vi "AlliGator Update Background Subtraction Indicators.vi"(8 "Error In":errorcluster, 10 "Decay Metadata":T1={"ROI Descriptor"={"Global Rectangle"=[], "Contours"=[]}, "ROI Center"={"X"=0, "Y"=0}, "Decay Background Subtraction Info"={"Laser Period"=0.0, "Gate Duration"=0.0, "Baseline Subtraction Method"=enum."Mean", "Background Definition Range"={"Min Gate"=0.0, "Max Gate"=0.0}, "Total Intensity w/o Bkgd Subtraction"=0.0, "Bkgd-subtracted Intensity (exp)"=0.0, "# Data Points"=0, "Background/Gate"=0.0, "Fitted Lifetime"=0.0, "Bkgd-subtracted Intensity (theo)"=0.0}, "Decay Reverted"=FALSE, "Decay Smoothened"=FALSE, "Decay Straightened"=FALSE, "Fitted Tau (Decay Straightening)"=0.0, "Decay Shift Parameters"={"Type"=enum."Default", "Shift"=0.0, "Threshold"=0.0, "Rotate"=FALSE}, "Decay Shifted"=FALSE, "Decay Extrapolated"=FALSE, "Decay Extrapolation Parameters"={"Additional Points"=0, "Head Fraction"=0.0, "Fitted Tau"=0.0, "Use Periodicity"=FALSE, "Use Cursors"=FALSE, "Tail Fraction"=0.0}, "Decay Normalized"=FALSE, "Fold Decay"=FALSE, "# Folds"=1} {"# Folds" min=1; "ROI Descriptor"."Contours"."Type" items=["No Selection", "Point", "Line", "Rectangle", "Oval", "Polygon", "Freehand Region", "Annulus", "Unused2", "Unused3", "Broken Line", "Freehand Line", "Rotated Rectangle"]}, 11 "AlliGator Ref":refnum<vi>) -> (0 "Error Out":errorcluster)   [LabVIEW 2021, in "AlliGator Decay Analysis.lvlib" / "AlliGator Decay Preprocessing.lvlib"]
doc: "Updates background subtraction indicators in the <B>Decay Graph</B> panel."
uses:
  AlliGator Decay Preprocessing.lvlib
  AlliGator Decay Metadata v3.ctl
  AlliGator Decay Background Subtraction Info.ctl
  AlliGator Baseline Subtraction Method.ctl
  Graphs/XY Graph/XY Graph Plot Shift Parameters.ctl
  Graphs/XY Graph/XY Graph Plot Shift Method.ctl
  AlliGator Decay Extrapolation Parameters.ctl
  AlliGator Settings List.ctl
  Variant/Variant to Data/Variant to Boolean.vi
  AlliGator Settings.lvlib
  Variant/Variant to Data/Variant to Data.lvlib
  Utilities/Utilities.lvlib
  AlliGator Phasor Graph.lvlib
  Graphs/XY Graph/XY Graph Add-Ons.lvlib
panel:
  out "Integrated Intensity":dbl
  out "Lifetime":dbl[unit]=nan
  out "Background/Gate":dbl
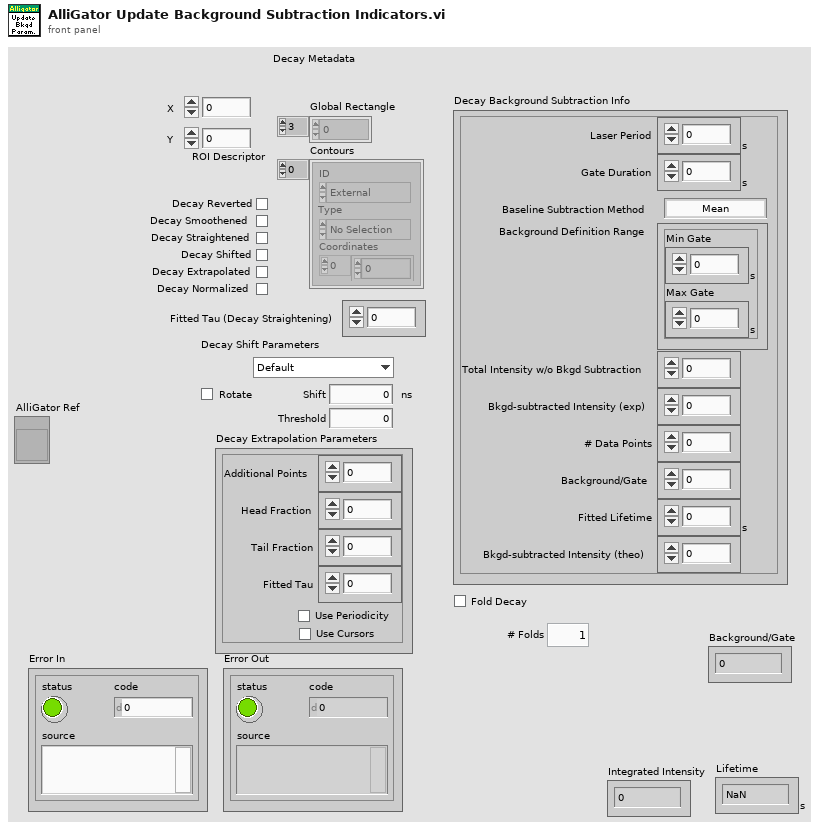
[diagram p1: front panel]
types:
  T1 = typedef "AlliGator Phasor Graph.lvlib/AlliGator Decay Metadata v3.ctl" = cluster{"ROI Descriptor":T2, "ROI Center":cluster{"X":i32, "Y":i32}, "Decay Background Subtraction Info":T3, "Decay Reverted":bool, "Decay Smoothened":bool, "Decay Straightened":bool, "Fitted Tau (Decay Straightening)":dbl, "Decay Shift Parameters":T5, "Decay Shifted":bool, "Decay Extrapolated":bool, "Decay Extrapolation Parameters":T7, "Decay Normalized":bool, "Fold Decay":bool, "# Folds":u32}
  T2 = typedef "ROI Descriptor" = cluster{"Global Rectangle":i32[], "Contours":cluster{"ID":enum32{"External", "Internal"}, "Type":u32, "Coordinates":i32[]}[]}
  T3 = typedef "AlliGator Decay Analysis.lvlib/AlliGator Decay Preprocessing.lvlib/AlliGator Decay Background Subtraction Info.ctl" = cluster{"Laser Period":dbl[unit], "Gate Duration":dbl[unit], "Baseline Subtraction Method":T4, "Background Definition Range":cluster{"Min Gate":dbl[unit], "Max Gate":dbl[unit]}, "Total Intensity w/o Bkgd Subtraction":dbl, "Bkgd-subtracted Intensity (exp)":dbl, "# Data Points":i32, "Background/Gate":dbl, "Fitted Lifetime":dbl[unit], "Bkgd-subtracted Intensity (theo)":dbl}
  T4 = typedef "AlliGator Decay Analysis.lvlib/AlliGator Decay Preprocessing.lvlib/AlliGator Baseline Subtraction Method.ctl" = enum16{"Mean", "Min", "Square Gated Single-Exponential", "File", "Constant"}
  T5 = typedef "XY Graph Add-Ons.lvlib/XY Graph Plot Shift Parameters.ctl" = cluster{"Type":T6, "Shift":dbl[unit], "Threshold":dbl, "Rotate":bool}
  T6 = typedef "XY Graph Add-Ons.lvlib/XY Graph Plot Shift Method.ctl" = enum16{"Default", "CFD", "Threshold", "Cross-Correlation"}
  T7 = typedef "AlliGator Decay Analysis.lvlib/AlliGator Decay Preprocessing.lvlib/AlliGator Decay Extrapolation Parameters.ctl" = cluster{"Additional Points":u32, "Head Fraction":dbl, "Fitted Tau":dbl, "Use Periodicity":bool, "Use Cursors":bool, "Tail Fraction":dbl}
  T8 = typedef "AlliGator Settings.lvlib/AlliGator Settings List.ctl" = enum16{"GUI:Visible Settings Tab", "GUI:Last Run Version", "Source Image:Use Image Histogram for Contrast", "Source Image:Low Count Pixels Rejection Options", "Source Image:High Count Pixels Rejection Options", "Source Image:Use Image Brightness", "Source Image:Blend Overlay with Image Background", "Source Image:Use Fixed ROI Diameter", "Source Image:ROI Diameter", "Source Image:ROI Center Color", "Source Image:Peak Threshold", "Source Image:Intensity Threshold", "Source Image:Image Binning Options", "Source Image:Image Smoothing Options", "Source Image:Image Histogram Active", "Source Image:Invert Binary Mask", "Source Image:Hot Pixel Removal", "Source Image:Overlay Analyzed ROI Center", "Source Image:Auto-Adjust Contrast", "Source Image:Histogram Lower Percentile", "Source Image:Histogram Upper Percentile", "Source Image:Save Source Image", "Source Image:Scale Bar Options", "Source Image:Image Resolution (Pixel Size)", "Data Information:Gate Width", "Data Information:Nanotime Gate Separation", "Data Information:Macrotime Gate Separation", "Data Information:Gate Step", "Data Information:# Gates", "Data Information:Gate Image Exposure", "Data Information:Gate Image Integration", "Data Information:Gates to Skip", "Data Information:Gates to Keep", "Data Information:Define Gates to", "Data Information:Channel Name", "Data Information:Available Channel Names", "Data Information:Channel Arithmetic", "Data Information:Background File Subtraction", "Data Information:Background File", "Data Information:Background Scaling Factor", "Data Information:Background Pile-up Correction", "Data Information:Background Pixel Well Capacity", "Data Information:Laser Period", "Data Information:SYNC Period", "Data Information:Pile-up Correction", "Data Information:Pixel Well Capacity", "Data Information:Dataset Scaling Factor", "Fluorescence Decay_Decay Pre-Processing:Reverse Gates", "Fluorescence Decay_Decay Pre-Processing:Verbose Decay Pre-Processing", "Fluorescence Decay_Decay Pre-Processing:Use Decay Pre-Processing", "Fluorescence Decay_Decay Pre-Processing:Background Subtraction", "Fluorescence Decay_Decay Pre-Processing:Background Definition Range", "Fluorescence Decay_Decay Pre-Processing:Baseline Subtraction Method", "Fluorescence Decay_Decay Pre-Processing:Operations Order", "Fluorescence Decay_Decay Pre-Processing:Smoothing Parameter", "Fluorescence Decay_Decay Pre-Processing:Shift Decay", "Fluorescence Decay_Decay Pre-Processing:Decay Shift Parameters", "Fluorescence Decay_Decay Pre-Processing:Fold Decay", "Fluorescence Decay_Decay Pre-Processing:# Folds", "Fluorescence Decay_Decay Pre-Processing:1-Normalize Decay", "Fluorescence Decay_Decay Pre-Processing:[0-1]-Normalize Decay", "Fluorescence Decay_Decay Pre-Processing:Smoothen Decay", "Fluorescence Decay_Decay Pre-Processing:Extrapolate Decay", "Fluorescence Decay_Decay Pre-Processing:Use Periodicity", "Fluorescence Decay_Decay Pre-Processing:Use Cursors", "Fluorescence Decay_Decay Pre-Processing:Tail Fraction", "Fluorescence Decay_Decay Pre-Processing:Head Fraction", "Fluorescence Decay_Decay Pre-Processing:Additional Points", "Fluorescence Decay_Decay Pre-Processing:Straighten Decay", "Fluorescence Decay_Decay Pre-Processing:Constant Background", "Fluorescence Decay_Decay Pre-Processing:Pixel-Normalize Decay", "Fluorescence Decay_Advanced Analysis:Extract IRF instead of Decay", "Fluorescence Decay_Advanced Analysis:IRF Extraction Options", "Fluorescence Decay_Advanced Analysis:IRF Optimization Options", "Fluorescence Decay_Advanced Analysis:Square Pulse Options", "Fluorescence Decay_Advanced Analysis:IRF Order", "Fluorescence Decay_Advanced Analysis:IRF Time Constants", "Fluorescence Decay_Advanced Analysis:Wavelet Analysis Options", "Fluorescence Decay_Advanced Analysis:Average Lifetime Options", "Fluorescence Decay_Fit Options:Fit Options", "Fluorescence Decay_Fit Options:Use Legacy Fitting Approach", "Fluorescence Decay_Fit Options:Use Data Information Laser Period", "Fluorescence Decay_Fit Parameters:Displayed Fit Parameters", "Fluorescence Decay_Fit Parameters:Fit Parameter Constraints", "Fluorescence Decay_Fit Parameters:Export Tabulated Results", "Fluorescence Decay_Fit Parameters:MLE Baseline Offset Type", "Fluorescence Decay_Fit Parameters:MLE Baseline Offset", "Fluorescence Decay_Fit Parameters:Guess Parameter Names", "Fluorescence Decay_Fit Parameters:Guess Parameter Values", "Fluorescence Decay_Fit Parameters:Guess Parameters Options", "Fluorescence Decay_Styles:Show Last Decay Only", "Fluorescence Decay_Styles:Decay Graph Color Array", "Fluorescence Decay:Decay Graph Active", "Fluorescence Decay Statistics:Min Peak Value", "Fluorescence Decay Statistics:Reject Low Decay Peak Pixels", "Fluorescence Decay Statistics:Reject High Decay Peak Pixels", "Fluorescence Decay Statistics:Max Peak Value", "Time Traces:Use File Timestamp", "Time Traces:Time Step", "Time Traces:Use Intensity Correction File", "Time Traces:Intensity Correction File", "Phasor Plot:Phasor Plot Smoothing Options", "Phasor Plot:Phasor Plot Size", "Phasor Plot:Phasor Plot Graphics Options", "Phasor Plot:Cumulative Phasor Plot", "Phasor Plot:Use Phasor Brightness", "Phasor Plot:Blend Overlay with Phasor Background", "Phasor Plot:Save Phasor Plot", "Phasor Plot:Show References", "Phasor Plot:Phasor Ratio Decay Range", "Phasor Plot:Exponential Fading", "Phasor Plot:Phasor Ratio Reference Colors", "Phasor Plot:Reference Radius", "Phasor Plot:Show Color Map Vertices", "Phasor Plot:Phasor Plot Active", "Phasor Plot:Phasor Ratio Color Map Type", "Phasor Plot:Phasor Ratio Color Map", "Phasor Plot:Phasor Ratio Display Range", "Phasor Plot:Selected Image ROI(s)", "Phasor Plot:All Image ROIs", "Phasor Plot:Selected Phasor Plot ROI(s)", "Phasor Plot:All Phasor Plot ROIs", "Phasor Plot:Phasor Ratio Color-Coded Quantity", "Phasor Plot:Store Phasor Harmonics", "Phasor Plot:Draw Reference Segment", "Phasor Plot:User-Defined Quantity", "Phasor Graph:Phasor Frequency", "Phasor Graph:Phasor Ratio Type", "Phasor Graph:Pixel-level Phasor Computation", "Phasor Graph:Save Phasor Graph", "Phasor Graph:Phasor Graph Active", "Phasor Graph:Phasor SDV Options", "Phasor Calibration:Use Backup Calibration if needed", "Phasor Graph:Define Shortest Lifetime as", "Phasor Calibration:Backup Calibration Type", "Phasor Calibration:Calibration Type", "Phasor Calibration:Calibration Lifetime", "Phasor Calibration:Calibration Map Algorithm", "Single-Exponential Phasor Locus (SEPL):Gate Parameters", "Single-Exponential Phasor Locus (SEPL):User-defined Gate", "Single-Exponential Phasor Locus (SEPL):User-defined IRF", "Single-Exponential Phasor Locus (SEPL):Phasor Parameters", "Single-Exponential Phasor Locus (SEPL):Decay & IRF Parameters", "Single-Exponential Phasor Locus (SEPL):Display Parameters", "Lifetime Analysis:Decay Analysis Parameters", "Lifetime Analysis:Lifetime Map Active", "Plugins:Python Settings", "Miscellaneous:Verbose Mode", "Miscellaneous:Beep after Script", "Miscellaneous:Saved Image File Format", "Miscellaneous:Exported Gate Image Settings", "Miscellaneous:Include Loading in Timing", "Miscellaneous:Verbose Settings Mode", "Miscellaneous:Histogram Options", "Miscellaneous:Beep on Error", "Miscellaneous:# Logical Processors Used", "Miscellaneous:ROI Description Max Characters", "Miscellaneous:Verbose Error Mode", "Miscellaneous:Transparent Mask Color"}
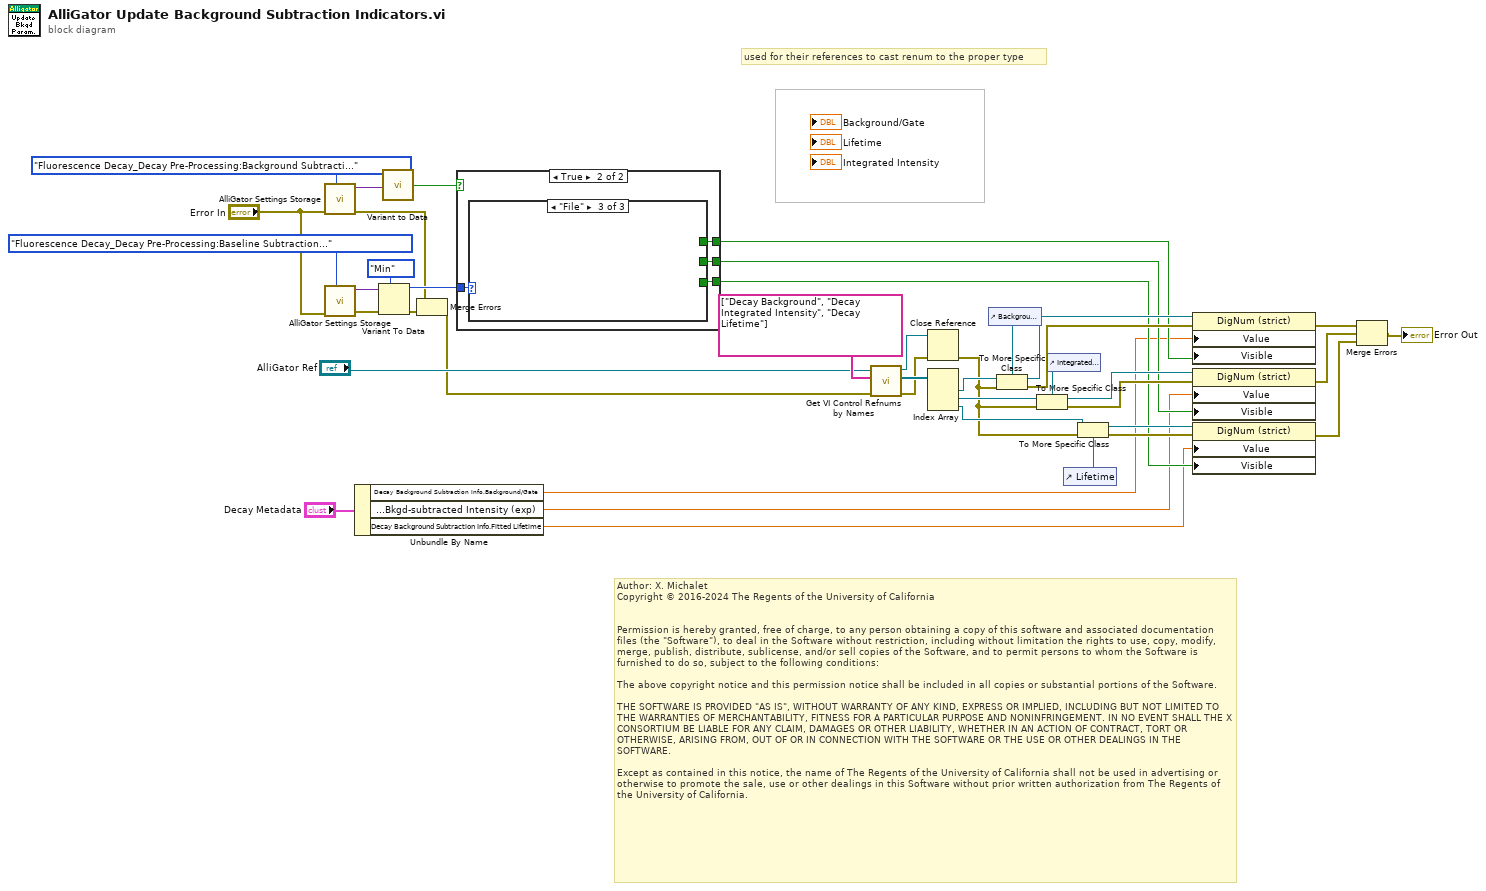
[diagram p0: block diagram]
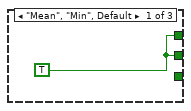
[diagram p3: hidden frame]
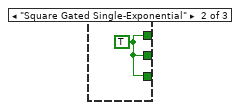
[diagram p4: hidden frame]
diagram:
  # "used for their references to cast renum to the proper type"
  # "Author: X. Michalet\nCopyright © 2016-2024 The Regents of the University of California\n \n\nPermission is hereby granted, free of charge, to any person obtaining a copy of this software and associated documentation files (the \"Software\"), to deal in the Software without restriction, including without limitation the rights to use, copy, modify, merge, publish, distribute, sublicense, and/or sell copies of the Software, and to permit persons to whom the Software is furnished to do so, subject to the following conditions:\n\nThe above copyright notice and this permission notice shall be included in all copies or substantial portions of the Software.\n\nTHE SOFTWARE IS PROVIDED \"AS IS\", WITHOUT WARRANTY OF ANY KIND, EXPRESS OR IMPLIED, INCLUDING BUT NOT LIMITED TO THE WARRANTIES OF MERCHANTABILITY, FITNESS FOR A PARTICULAR PURPOSE AND NONINFRINGEMENT. IN NO EVENT SHALL THE X CONSORTIUM BE LIABLE FOR ANY CLAIM, DAMAGES OR OTHER LIABILITY, WHETHER IN AN ACTION OF CONTRACT, TORT OR OTHERWISE, ARISING FROM, OUT OF OR IN CONNECTION WITH THE SOFTWARE OR THE USE OR OTHER DEALINGS IN THE SOFTWARE.\n\nExcept as contained in this notice, the name of The Regents of the University of California shall not be used in advertising or otherwise to promote the sale, use or other dealings in this Software without prior written authorization from The Regents of the University of California."
  n1 = call "AlliGator Settings Storage.vi"("AlliGator Settings List"=AlliGator_Settings_List."Fluorescence Decay_Decay Pre-Processing:Background Subtraction", "Error In"="Error In") -> ("Error Out"=w5:errorcluster, "Variant Data out"=w41:variant)  [unwired: 8 in]
  n2 = call "AlliGator Settings Storage.vi"("AlliGator Settings List"=AlliGator_Settings_List."Fluorescence Decay_Decay Pre-Processing:Baseline Subtraction Method", "Error In"="Error In") -> ("Error Out"=w38:errorcluster, "Variant Data out"=w37:variant)  [unwired: 8 in]
  n3 = Unbundle By Name("Decay Metadata") -> ("Decay Background Subtraction Info.Background/Gate"=w10:dbl, "Decay Background Subtraction Info.Bkgd-subtracted Intensity (exp)"=w9:dbl, "Decay Background Subtraction Info.Fitted Lifetime"=w8:dbl[unit])
  n4 = Variant To Data(error in=w38, type=AlliGator_Baseline_Subtraction_Method."Min" ("Baseline Subtraction Method"), Variant=w37) -> (data=w34:T4, error out=w7:errorcluster)
  n5 = call-poly "Variant to Data.vi"("Variant"=w41) -> ("Value"=w35:bool)  [unwired: 8 in]
  n6 = Merge Errors(w5, w7) -> (w6:errorcluster)
  n7 = case shown="True" w35 {
    selector: w35 -> [w42 _]
    tunnel: [w42 w45] -> w13
    tunnel: [w42 w44] -> w12
    tunnel: [w42 w43] -> w11
    tunnel: w34 -> [_ w46]
    frame False {
    }
    frame True {
      n8 = case shown="\"File\"" w46 {
        tunnel: [w47 w48 _] -> w45
        tunnel: [w47 w48 _] -> w44
        tunnel: [_ w48 _] -> w43
        frame "Mean", "Min", Default {
          w47 = TRUE
        }
        frame "Square Gated Single-Exponential" {
          w48 = TRUE
        }
        frame "File" {
        }
      }
    }
  }
  n9 = call "Get VI Control Refnums by Names.vi"("error in"=w6, "Control Labels"=string[] ["Decay Background", "Decay Integrated Intensity", "Decay Lifetime"], "VI  Ref"="AlliGator Ref") -> ("error out"=w30:errorcluster, "Ctl Refnums"=w32:refnum<vi>[], "VI  Ref (out)"=w29:refnum<vi>)  [unwired: 5 in, 1 out]
  n10 = Close Reference(reference=w29, error in (no error)=w30) -> (error out=w25:errorcluster)
  n11 = Index Array(array=w32) -> (element #1=w27:refnum<vi>, element #2=w31:refnum<vi>, element #3=w26:refnum<vi>)  [unwired: 3 in]
  n12 = control-ref of="Background/Gate"() -> (w24:refnum<vi>)
  n13 = To More Specific Class(target class=w24, reference=w27, error in=w25) -> (specific class reference=w23:refnum<vi>, error out=w18:errorcluster)
  n14 = control-ref of="Integrated Intensity"() -> (w22:refnum<vi>)
  n15 = To More Specific Class(target class=w22, reference=w31, error in=w25) -> (specific class reference=w21:refnum<vi>, error out=w17:errorcluster)
  n16 = control-ref of="Lifetime"() -> (w20:refnum<vi>)
  n17 = To More Specific Class(target class=w20, reference=w26, error in=w25) -> (specific class reference=w19:refnum<vi>, error out=w16:errorcluster)
  n18 = property class="DigNum (strict)"(reference=w23, error in=w18, "Value"=w10, "Visible"=w13) -> (error out=w4:errorcluster)  [unwired: 1 out]
  n19 = property class="DigNum (strict)"(reference=w21, error in=w17, "Value"=w9, "Visible"=w12) -> (error out=w3:errorcluster)  [unwired: 1 out]
  n20 = property class="DigNum (strict)"(reference=w19, error in=w16, "Value"=w8, "Visible"=w11) -> (error out=w2:errorcluster)  [unwired: 1 out]
  n21 = Merge Errors(w4, w3, w2) -> (→"Error Out":errorcluster)
